vi "Write From String Delimiter.vi"(8 "error in (no error)":errorcluster, 10 "From String Delimiter":string=",", 11 "Abs_Array in":refnum<class "Abs_Array.lvclass">) -> (0 "error out":errorcluster, 3 "Abs_Array out":refnum<class "Abs_Array.lvclass">)   [LabVIEW 2021, in "Abs_Array.lvclass"]
uses:
  Abs_Array.lvclass
  Abs_Array.lvclass/Abs_Array.ctl
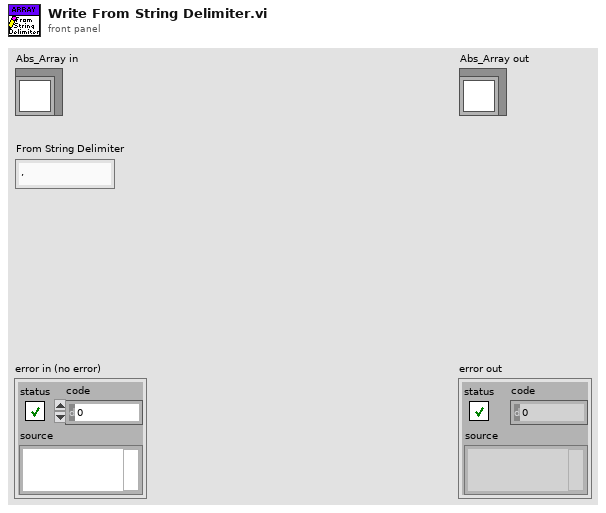
[diagram p1: front panel]
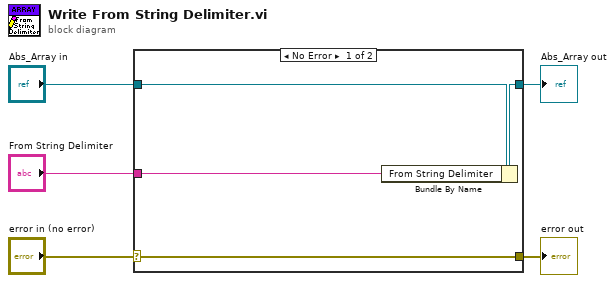
[diagram p0: block diagram]
diagram:
  n1 = case shown="No Error" "error in (no error)" {
    selector: "error in (no error)" -> [w9 w10]
    tunnel: [w9 w10] -> w4
    tunnel: [w7 w11] -> w2
    tunnel: "Abs_Array in" -> [w8 w11]
    tunnel: "From String Delimiter" -> [w6 _]
    frame No Error {
      n2 = Bundle By Name(cluster=w8, "From String Delimiter"=w6) -> (w7:refnum<class "Abs_Array.lvclass">)
    }
    frame Error {
    }
  }
  "error out" <- w4
  "Abs_Array out" <- w2
